vi "Filter_uA_low_range_30u.vi"(7 "Frequency":dbl=66.676136425152, 9 "uA_calib_0":dbl=1.5 format="%#_13g", 10 "mA/uA":bool, 11 "in":dbl[](array[numeric])) -> (3 "out":dbl[](array[numeric]))   [LabVIEW 2015]
panel:
  out "sum":dbl
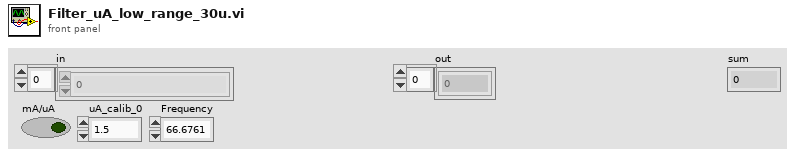
[diagram p1: front panel]
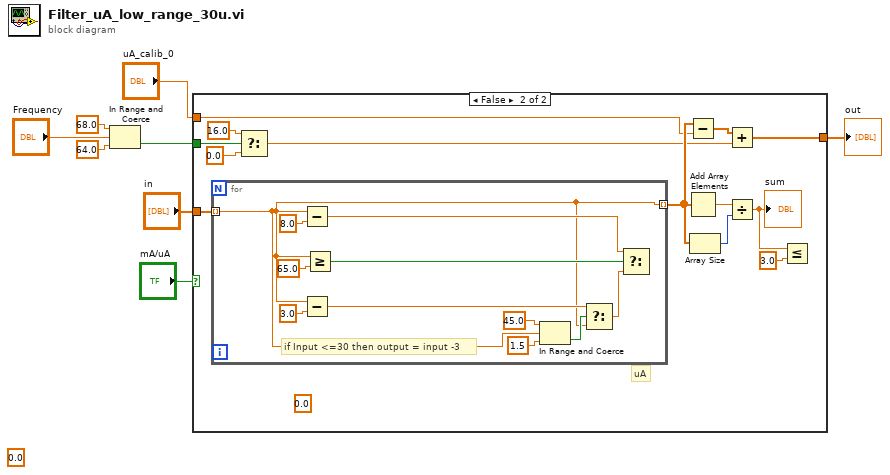
[diagram p0: block diagram]
diagram:
  (unwired) 0.0
  n1 = In Range and Coerce(upper limit=68.0, x="Frequency", lower limit=64.0) -> (In Range?=w1:bool)  [unwired: 1 out]
  n2 = case shown="False" "mA/uA" {
    tunnel: "in" -> [w9 w22]
    tunnel: "uA_calib_0" -> [_ w16]
    tunnel: [w9 w13] -> w6
    tunnel: w1 -> [_ w15]
    frame True {
      # "mA"
    }
    frame False {
      (unwired) 0.0 ("f")
      # "uA"
      n3 = for {
        tunnel: w22 -> [w23] mode=indexing
        tunnel: [w23] -> w21 mode=indexing
        # "if Input <=30 then output = input -3"
        n4 = Subtract(x=w23, y=8.0) -> (x-y=w25:dbl)
        n5 = Subtract(x=w23, y=3.0) -> (x-y=w33:dbl)
        n6 = Greater Or Equal?(x=w23, y=65.0) -> (x >= y?=w27:bool)
        n7 = In Range and Coerce(upper limit=45.0 ("y"), x=w23, lower limit=1.5) -> (In Range?=w30:bool)  [unwired: 1 out]
        n8 = Select(t=w33, s=w30, f=w23) -> (s? t:f=w24:dbl)
        n9 = Select(t=w25, s=w27, f=w24) -> ()  [unwired: 1 out]
      }
      n10 = Select(t=16.0, s=w15, f=0.0) -> (s? t:f=w12:dbl)
      n11 = Subtract(x=w21, y=w16) -> (x-y=w14:dbl[])
      n12 = Add Array Elements(numeric array=w21) -> (sum=w20:dbl)
      n13 = Array Size(array=w21) -> (size(s)=w19:i32)
      n14 = Add(x=w14, y=w12) -> (x+y=w13:dbl[])
      n15 = Divide(x=w20, y=w19) -> (x/y=w17:dbl)
      "sum" <- w17
      n16 = Less Or Equal?(x=w17, y=3.0) -> ()  [unwired: 1 out]
    }
  }
  "out" <- w6
